vi "Configure Output Channels.vi"(8 "error in (no error)":errorcluster, 10 "Output Channel Refs":T4[](array[typedef]) format="%.0x", 11 "Device Ref in":T4 format="%.0x") -> (0 "error out":errorcluster, 1 "Output Channels":T3 {"Output Block Data Refs"."Data Reference" format="%.0x"}, 2 "RT FIFO Write out":refnum<k33>, 3 "Device Ref out":T4 format="%.0x")   [LabVIEW 2015, in "Shared Variable Custom Device.lvlib"]
doc: "Get the Output channels' block references and the RT FIFO Write."
uses:
  Shared Variable Custom Device.lvlib
  <vilib>/NI Veristand/Custom Device API/Custom Device Item Ref.ctl
  <vilib>/NI Veristand/Custom Device API/Block Data Reference.ctl
  <vilib>/NI Veristand/Custom Device API/Data Reference.ctl
  <vilib>/NI Veristand/Custom Device API/Data Access Type.ctl
  <vilib>/NI Veristand/Custom Device API/Custom Device API.lvlib
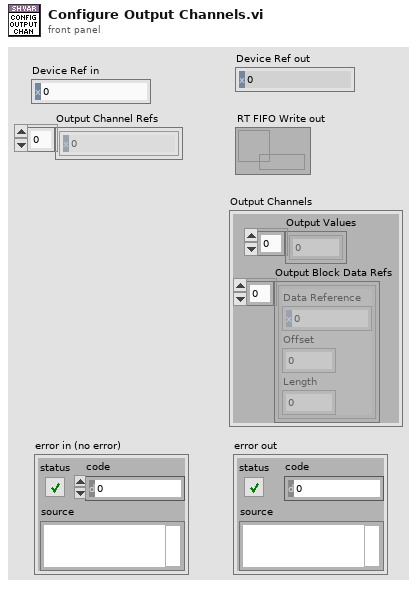
[diagram p1: front panel]
types:
  T1 = typedef "Custom Device API.lvlib/Block Data Reference.ctl" = cluster{"Data Reference":T2, "Offset":u64, "Length":u64}
  T2 = typedef "Custom Device API.lvlib/Data Reference.ctl" = i32
  T3 = cluster{"Output Values":dbl[], "Output Block Data Refs":T1[]}
  T4 = typedef "Custom Device API.lvlib/Custom Device Item Ref.ctl" = u64
  T5 = typedef "Custom Device API.lvlib/Data Access Type.ctl" = enum16{"Read", "Write"}
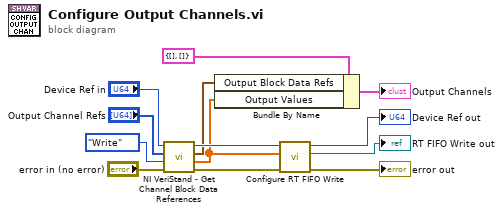
[diagram p0: block diagram]
diagram:
  n1 = call <vilib>:"NI VeriStand - Get Channel Block Data References.vi"("error in (no error)"="error in (no error)", "Access"=Data_Access_Type."Write", "Channel Refs"="Output Channel Refs", "Device Ref in"="Device Ref in") -> ("error out"=w12:errorcluster, "Values Array"=w5:dbl[], "Block Data Refs"=w4:T1[], "Device Ref out"=w13:T4)  [unwired: 4 in]
  n2 = Bundle By Name(cluster=T3 {"Output Values"=[], "Output Block Data Refs"=[]} ("Output Channels"), "Output Block Data Refs"=w4, "Output Values"=w5) -> (→"Output Channels":T3)
  n3 = call "Configure RT FIFO Write.vi"("error in (no error)"=w12, "Ouput Values Array"=w5, "Device Ref in"=w13) -> ("error out"=→"error out":errorcluster, "RT FIFO Write out"=→"RT FIFO Write out":refnum<k33>, "Device Ref out"=→"Device Ref out":T4)  [unwired: 6 in]
